vi "Array Create.vi"   [LabVIEW 2015, in "MDSplus.lvlib"]
uses:
  <vilib>/MDSplus/Library/MDSplus.lvlib
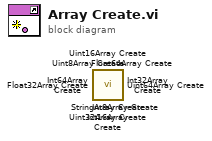
[diagram p0: block diagram]
diagram:
  n1 = call <vilib>:"StringArray Create.vi"() -> ()  [unwired: 10 in, 2 out]
  n2 = call <vilib>:"Float64Array Create.vi"() -> ()  [unwired: 10 in, 2 out]
  n3 = call <vilib>:"Float32Array Create.vi"() -> ()  [unwired: 10 in, 2 out]
  n4 = call <vilib>:"Uint64Array Create.vi"() -> ()  [unwired: 10 in, 2 out]
  n5 = call <vilib>:"Uint32Array Create.vi"() -> ()  [unwired: 10 in, 2 out]
  n6 = call <vilib>:"Uint16Array Create.vi"() -> ()  [unwired: 10 in, 2 out]
  n7 = call <vilib>:"Uint8Array Create.vi"() -> ()  [unwired: 10 in, 2 out]
  n8 = call <vilib>:"Int64Array Create.vi"() -> ()  [unwired: 10 in, 2 out]
  n9 = call <vilib>:"Int32Array Create.vi"() -> ()  [unwired: 10 in, 2 out]
  n10 = call <vilib>:"Int16Array Create.vi"() -> ()  [unwired: 10 in, 2 out]
  n11 = call <vilib>:"Int8Array Create.vi"() -> ()  [unwired: 10 in, 2 out]
